vi "GetSelecteControlRef.vi"(0 "index":i32, 1 "Ref Cluster":T1) -> (14 "Control out":refnum<vi>)   [LabVIEW 2018]
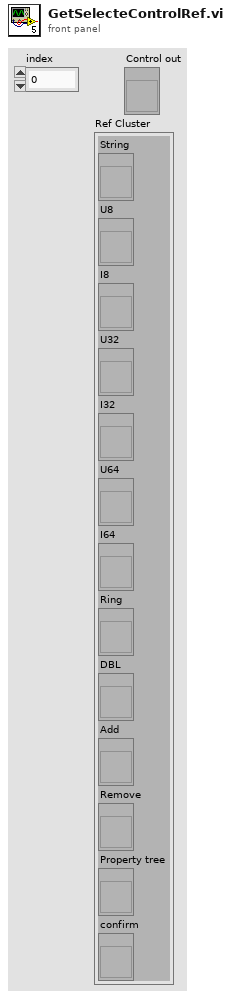
[diagram p1: front panel]
types:
  T1 = cluster{"String":refnum<vi>, "U8":refnum<vi>, "I8":refnum<vi>, "U32":refnum<vi>, "I32":refnum<vi>, "U64":refnum<vi>, "I64":refnum<vi>, "Ring":refnum<vi>, "DBL":refnum<vi>, "Add":refnum<vi>, "Remove":refnum<vi>, "Property tree":refnum<vi>, "confirm":refnum<vi>}
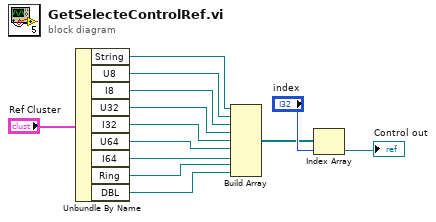
[diagram p0: block diagram]
diagram:
  n1 = Unbundle By Name("Ref Cluster") -> ("String"=w10:refnum<vi>, "U8"=w9:refnum<vi>, "I8"=w8:refnum<vi>, "U32"=w7:refnum<vi>, "I32"=w6:refnum<vi>, "U64"=w5:refnum<vi>, "I64"=w4:refnum<vi>, "Ring"=w3:refnum<vi>, "DBL"=w13:refnum<vi>)
  n2 = Build Array(w10, w9, w8, w7, w6, w5, w4, w3, w13) -> (w2:refnum<vi>[])
  n3 = Index Array(array=w2, index="index") -> (element=→"Control out":refnum<vi>)
